vi "Parse Controls.vi"(8 "error in (no error)":errorcluster, 10 "VI Type":T1(ring), 11 "Controls[]":refnum<vi>[](array[refnum])) -> (0 "error out":errorcluster, 3 "Control Names":string[](array[string]))   [LabVIEW 2016]
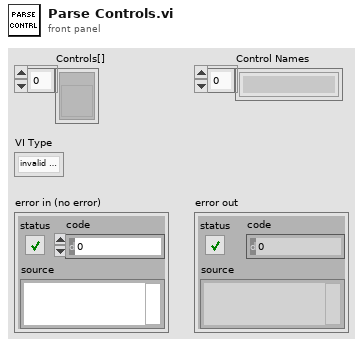
[diagram p1: front panel]
types:
  T1 = enum32{"invalid VI type", "Standard VI", "Control VI", "Global VI", "Polymorphic VI", "Configuration VI", "SubSystem", "Facade VI", "Method VI", "Statechart Diagram VI"}
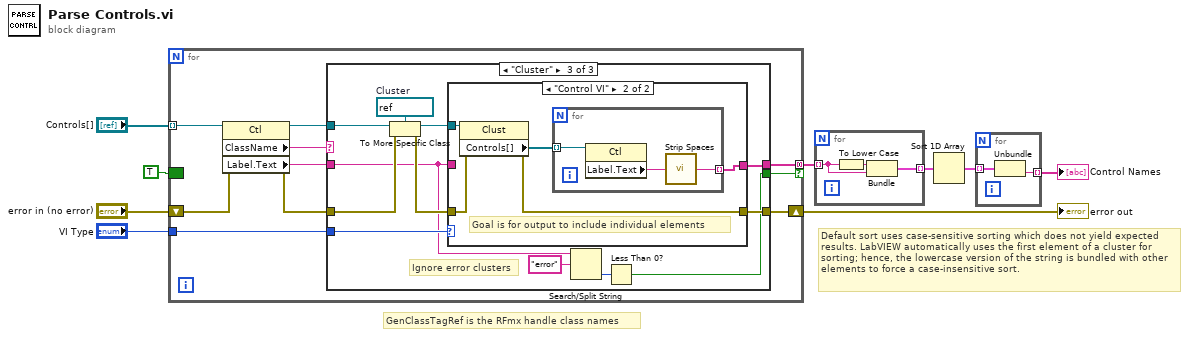
[diagram p0: block diagram]
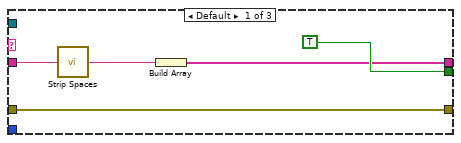
[diagram p2: hidden frame]
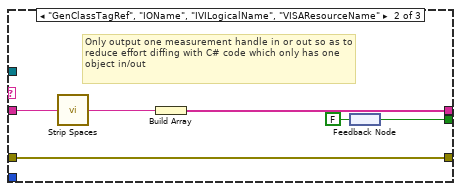
[diagram p3: hidden frame]
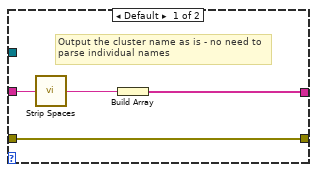
[diagram p4: hidden frame]
diagram:
  # "Default sort uses case-sensitive sorting which does not yield expected results. LabVIEW automatically uses the first element of a cluster for sorting; hence, the lowercase version of the string is bundled with other elements to force a case-insensitive sort."
  # "GenClassTagRef is the RFmx handle class names"
  n1 = for {
    tunnel: "Controls[]" -> [w19] mode=indexing
    shift-right: [w14] -> w7
    shift-left: "error in (no error)" -> [w17]
    tunnel: [w12] -> w5 mode=concatenating if=w11
    tunnel: "VI Type" -> [w10]
    border: TRUE -> [_]
    n2 = property class="Ctl"(reference=w19, error in=w17) -> (reference out=w18:refnum<vi>, error out=w15:errorcluster, "ClassName"=w16:string, "Label.Text"=w13:string)
    n3 = case shown="\"Cluster\"" w16 {
      tunnel: w18 -> [_ _ w42]
      tunnel: w15 -> [w24 w30 w40]
      tunnel: [w24 w30 w37] -> w14
      tunnel: w13 -> [w21 w28 w31]
      tunnel: [TRUE w26 w34] -> w11
      tunnel: [w22 w29 w33] -> w12
      tunnel: w10 -> [_ _ w32]
      frame Default {
        n4 = call "Strip Spaces.vi"("String In"=w21) -> ("result string"=w20:string)  [unwired: 14 in]
        n5 = Build Array(w20) -> (w22:string[])
      }
      frame "GenClassTagRef", "IOName", "IVILogicalName", "VISAResourceName" {
        # "Only output one measurement handle in or out so as to reduce effort diffing with C# code which only has one object in/out"
        n6 = call "Strip Spaces.vi"("String In"=w28) -> ("result string"=w27:string)  [unwired: 14 in]
        n7 = Build Array(w27) -> (w29:string[])
        n8 = feedback-in #1(FALSE) -> ()
        n9 = feedback #1() -> (w26:bool)
      }
      frame "Cluster" {
        w39 = refnum<vi> refnum  # Cluster
        # "Ignore error clusters"
        n10 = To More Specific Class(target class=w39, reference=w42, error in=w40) -> (specific class reference=w41:refnum<vi>, error out=w38:errorcluster)
        n11 = case shown="\"Control VI\"" w32 {
          tunnel: w41 -> [_ w51]
          tunnel: w38 -> [w46 w50]
          tunnel: [w46 w49] -> w37
          tunnel: [w45 w48] -> w33
          tunnel: w31 -> [w44 _]
          frame Default {
            # "Output the cluster name as is - no need to parse individual names"
            n12 = call "Strip Spaces.vi"("String In"=w44) -> ("result string"=w43:string)  [unwired: 14 in]
            n13 = Build Array(w43) -> (w45:string[])
          }
          frame "Control VI" {
            # "Goal is for output to include individual elements"
            n14 = property class="Clust"(reference=w51, error in=w50) -> (error out=w49:errorcluster, "Controls[]"=w47:refnum<vi>[])  [unwired: 1 out]
            n15 = for {
              tunnel: w47 -> [w54] mode=indexing
              tunnel: [w52] -> w48 mode=indexing
              n16 = property class="Ctl"(reference=w54) -> ("Label.Text"=w53:string)  [unwired: 1 in, 2 out]
              n17 = call "Strip Spaces.vi"("String In"=w53) -> ("result string"=w52:string)  [unwired: 14 in]
            }
          }
        }
        n18 = Search/Split String(string=w31, search string/char (-)="error") -> (offset of match=w35:i32)  [unwired: 1 in, 2 out]
        n19 = Less Than 0?(x=w35) -> (x < 0?=w34:bool)
      }
    }
  }
  "error out" <- w7
  n20 = for {
    tunnel: w5 -> [w57] mode=indexing
    tunnel: [w55] -> w4 mode=indexing
    n21 = To Lower Case(string=w57) -> (all lower case string=w56:string)
    n22 = Bundle(w56, "result string"=w57) -> (w55:cluster{string, "result string":string})  [unwired: 1 in]
  }
  n23 = Sort 1D Array(array=w4) -> (sorted array=w3:cluster{string, "result string":string}[])
  n24 = for {
    tunnel: w3 -> [w59] mode=indexing
    tunnel: [w58] -> w2 mode=indexing
    n25 = Unbundle(w59) -> ("result string"=w58:string)  [unwired: 1 out]
  }
  "Control Names" <- w2
